vi "SendMissionObstacleIDs.vi"(6 "Loop counter":i32, 8 "error in (no error)":errorcluster, 9 "# of Missions":i32, 10 "Obstacle Arrays Cluster":T1 {"Readable Obstacles"."Obstacle Array"."North" format="%#_10f"; "Readable Obstacles"."Obstacle Array"."East" format="%#_8f"}, 11 "NetworkStreamWriter in":refnum<class "NetworkStreamWriter.lvclass">) -> (0 "error out":errorcluster, 2 "Sending IDs?":bool, 3 "NetworkStreamWriter out":refnum<class "NetworkStreamWriter.lvclass">)   [LabVIEW 2013]
doc: "For the first 40 loop cycles this VI will wend the current mission and obstacle IDs to Main. These will be used to check against the IDs that Main has stored. If they don't match, Main will send its obstacles and missions back to the OCU to reorient the OCU. We want the missions and obstacles on the OCU to match those on the boat.\n\nEric Schneider, August 2014"
uses:
  RIO-OCU_Comm/NetworkStreams/Writer/NetworkStreamWriter.lvclass
  TypeDef/obstacle_arrays.ctl
  cRIO_Code/Logic/Classes/Obstacle/Obstacle.lvclass
  cRIO_Code/Data/TypeDefs/ObstacleDescription.ctl
  cRIO_Code/Data/TypeDefs/UTM Location.ctl
  CommandMessages.ctl
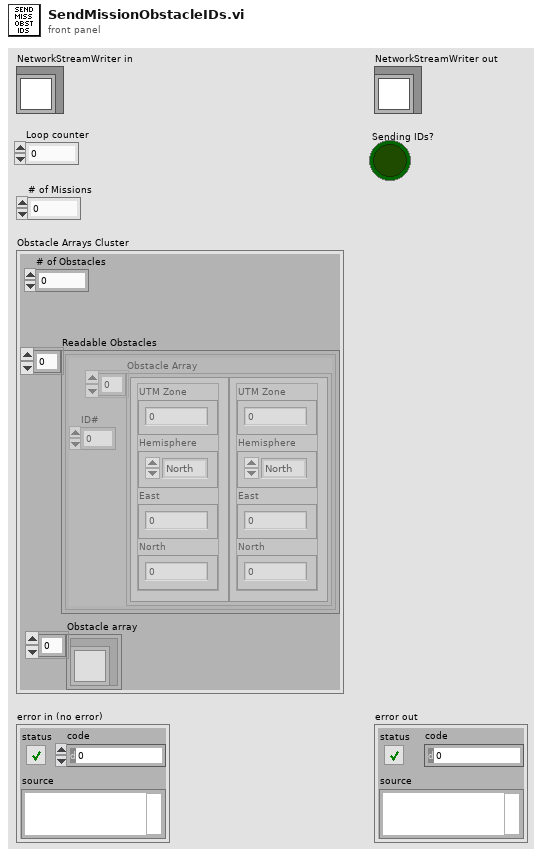
[diagram p1: front panel]
types:
  T1 = typedef "obstacle_arrays.ctl" = cluster{"# of Obstacles":i32, "Obstacle array":refnum<class "Obstacle.lvclass">[], "Readable Obstacles":T2[]}
  T2 = typedef "ObstacleDescription.ctl" = cluster{"ID#":i32, "Obstacle Array":T3[]}
  T3 = typedef "UTM Location.ctl" = cluster{"UTM Zone":dbl, "Hemisphere":enum16{"North", "South"}, "East":dbl, "North":dbl}
  T4 = typedef "CommandMessages.ctl" = enum16{"Pass", "OverrideMode", "Add mission", "Delete mission", "Add obstacle", "Delete obstacle", "Change constants", "Check mission ID", "Check obstacle ID"}
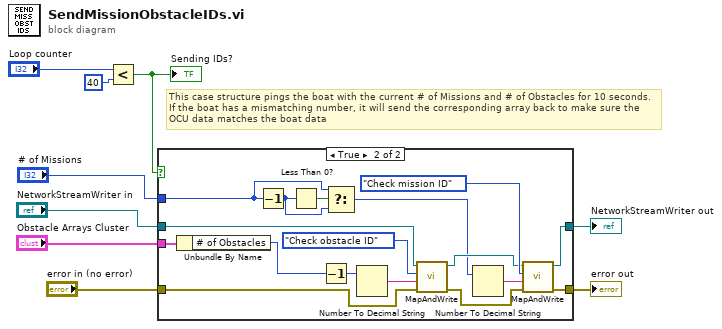
[diagram p0: block diagram]
diagram:
  # "This case structure pings the boat with the current # of Missions and # of Obstacles for 10 seconds. If the boat has a mismatching number, it will send the corresponding array back to make sure the OCU data matches the boat data"
  n1 = Less?(x="Loop counter", y=40) -> (x < y?=w8:bool)
  "Sending IDs?" <- w8
  n2 = case shown="True" w8 {
    tunnel: "error in (no error)" -> [w10 w18]
    tunnel: "NetworkStreamWriter in" -> [w11 w28]
    tunnel: "Obstacle Arrays Cluster" -> [_ w27]
    tunnel: [w10 w26] -> w4
    tunnel: [w11 w25] -> w5
    tunnel: "# of Missions" -> [_ w14]
    frame False {
    }
    frame True {
      n3 = Unbundle By Name(w27) -> ("# of Obstacles"=w12:i32)
      n4 = Decrement(x=w14) -> (x-1=w15:i32)
      n5 = Less Than 0?(x=w15) -> (x < 0?=w16:bool)
      n6 = Decrement(x=w12) -> (x-1=w21:i32)
      n7 = Select(t=w14, s=w16, f=w15) -> (s? t:f=w13:i32)
      n8 = Number To Decimal String(number=w21) -> (decimal integer string=w20:string)  [unwired: 1 in]
      n9 = call "MapAndWrite.vi"("error in (no error)"=w18, "String_Cast_of_Info"=w20, "Commands"=CommandMessages."Check obstacle ID", "NetworkStreamWriter in"=w28) -> ("error out"=w17:errorcluster, "NetworkStreamWriter out"=w22:refnum<class "NetworkStreamWriter.lvclass">)  [unwired: 2 in]
      n10 = Number To Decimal String(number=w13) -> (decimal integer string=w19:string)  [unwired: 1 in]
      n11 = call "MapAndWrite.vi"("error in (no error)"=w17, "String_Cast_of_Info"=w19, "Commands"=CommandMessages."Check mission ID", "NetworkStreamWriter in"=w22) -> ("error out"=w26:errorcluster, "NetworkStreamWriter out"=w25:refnum<class "NetworkStreamWriter.lvclass">)  [unwired: 2 in]
    }
  }
  "NetworkStreamWriter out" <- w5
  "error out" <- w4
